vi "clientAttachBroadcast.vi"(8 "error in (no error)":errorcluster, 11 "SM1000-control in":T1) -> (0 "error out":errorcluster, 2 "piClientId":i32, 3 "SM1000-control out":T1)   [LabVIEW 2013, in "SLMControl.lvlib" / "SM1000.lvclass"]
doc: "Establish a connection to receive broadcast messages.\n\nThis method is used by a client application to establish a connection to the broadcast mechanism of the EC1000. Once connected, a client may receive broadcast messages from all EC1000 modules on the network. The messages contain information about the broadcasting module including the name, internet IP address, and other relevant data. This data is retrieved through the use of 'getBroadcastData'."
uses:
  SM1000.lvclass
  Object-reference.ctl
  SM1000.lvclass/SM1000.ctl
  Custom-errors.ctl
  C:/Users/vangeste/Desktop/2015-06-02 - SLM - MAIF/HC-HardwareCharacterization/Sources/SM1000/LECBroadcast.dll
  HC-HardwareCharacterization/Sources/SM1000/LECBroadcast.dll
  DOTNET-error-int.vi
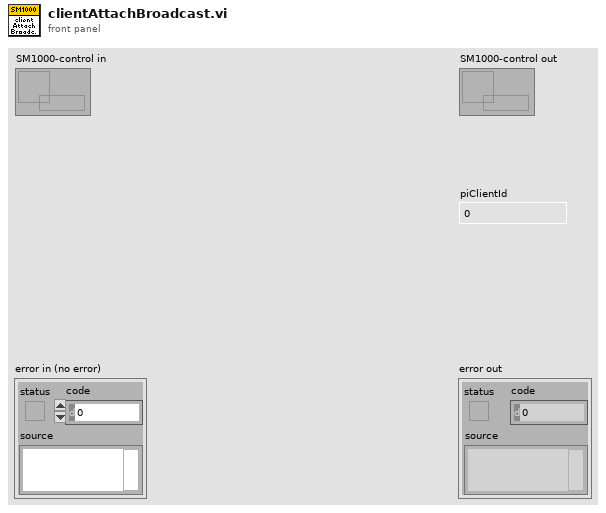
[diagram p1: front panel]
types:
  T1 = typedef "SLMControl.lvlib/SM1000.lvclass/Object-reference.ctl" = refnum<data-value>
  T2 = typedef "SLMControl.lvlib/SM1000.lvclass/Custom-errors.ctl" = enum16{"No error", "Not implemented", "Command not recognized", "Invalid input", "No connection", "Timeout", "Resource not loaded"}
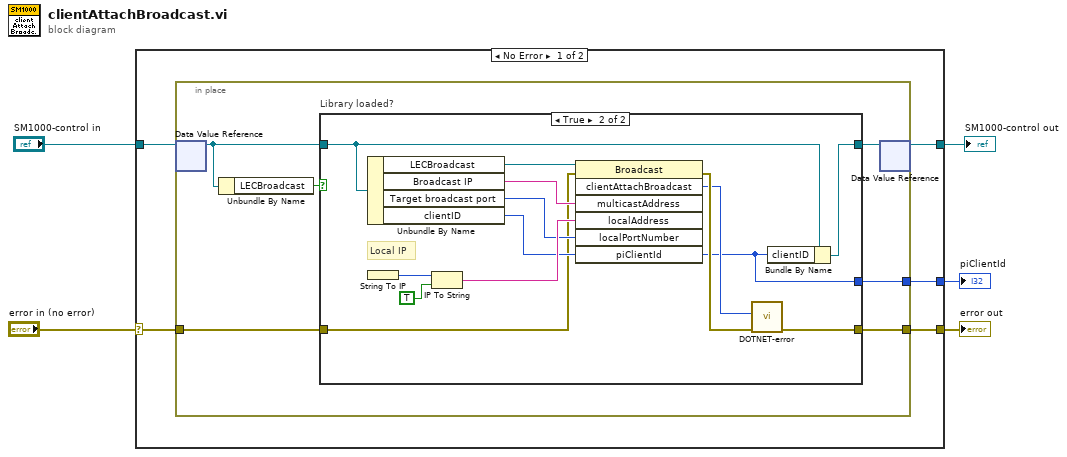
[diagram p0: block diagram]
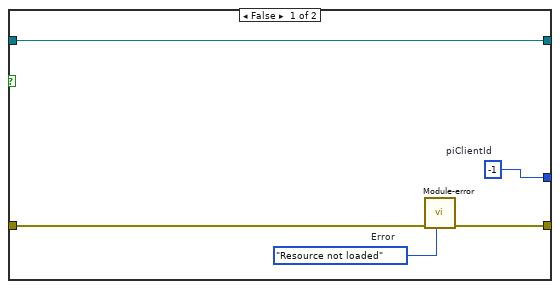
[diagram p2: hidden frame]
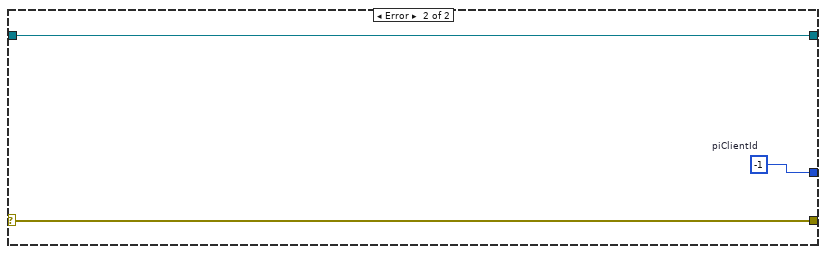
[diagram p3: hidden frame]
diagram:
  n1 = case shown="No Error" "error in (no error)" {
    selector: "error in (no error)" -> [w8 w38]
    tunnel: [w7 w38] -> w4
    tunnel: [w9 w37] -> w2
    tunnel: "SM1000-control in" -> [w10 w37]
    tunnel: [w6 w36] -> w1
    frame No Error {
      n2 = in-place {
        in-place-border: w8 -> [w16]
        in-place-border: [w13] -> w7
        in-place-border: [w11] -> w6
        n3 = in-place-dvr #1(w10) -> (w14:refnum<class "SM1000.lvclass">)  [unwired: 1 out]
        n4 = Unbundle By Name(w14) -> ("LECBroadcast"=w15:bool)
        n5 = case "Library loaded?" shown="True" w15 {
          tunnel: w16 -> [w21 w27]
          tunnel: w14 -> [w19 w35]
          tunnel: [w20 w33] -> w13
          tunnel: [w19 w24] -> w12
          tunnel: [w18 w23] -> w11
          frame False {
            w18 = -1  # piClientId
            w17 = Custom-errors."Resource not loaded"  # Error
            n6 = call "Module-error.vi"("Error"=w17, "error in (no error)"=w21) -> ("error out"=w20:errorcluster)  [unwired: 9 in]
          }
          frame True {
            # "Local IP"
            n7 = Unbundle By Name(w35) -> ("LECBroadcast"=w32:refnum<k24>, "Broadcast IP"=w31:string, "Target broadcast port"=w29:i32, "clientID"=w28:i32)
            n8 = String To IP() -> (0:w34:u32)  [unwired: 1 in]
            n9 = IP To String(1:TRUE, 2:w34) -> (0:w30:string)
            n10 = invoke class="Broadcast" method="clientAttachBroadcast"(reference=w32, error in=w27, "multicastAddress"=w31, "localAddress"=w30, "localPortNumber"=w29, "piClientId"=w28) -> (error out=w26:errorcluster, "clientAttachBroadcast"=w25:u32, "piClientId"=w23:i32)  [unwired: 1 in, 4 out]
            n11 = call-poly "DOTNET-error.vi"("error in (no error)"=w26, "Retun code"=w25) -> ("error out"=w33:errorcluster)  [unwired: 9 in]
            n12 = Bundle By Name(cluster=w35, "clientID"=w23) -> (w24:refnum<class "SM1000.lvclass">)
          }
        }
        n13 = in-place-dvr #1(w12) -> (w9:T1)  [unwired: 1 out]
      }
    }
    frame Error {
      w36 = -1  # piClientId
    }
  }
  "error out" <- w4
  "SM1000-control out" <- w2
  "piClientId" <- w1
